vi "Shell and Tube Heat Exchanger 3.vi"() -> ()   [LabVIEW 2017]
uses:
  <vilib>/addons/control/pid/pid.llb/PID Control Input Filter (DBL).vi
  <vilib>/addons/control/pid/pid.llb/PID Advanced (DBL).vi
  <vilib>/addons/control/pid/NI_PID_pid.lvlib
panel:
  out "Makeup Flowrate":dbl caption="L/min"
  out "Makeup Temperature":dbl caption="C"
  in  "Pump Switch":bool
  out "Water Outlet Temperature":dbl=22.816489944987293 format="%.1f"
  in  "Flowrate Setpoint (GPM)":dbl=40.0 min=0.0 max=50.0 format="%.2f"
  out "Water Flowrate":dbl=-0.0005338564515105265 format="%.2f"
  out "Flow Control Valve":dbl(slide)=100.0 scale=0.0..100.0
  in  "Manual Control Override (Flow)":bool=TRUE
  in  "Set Manual Valve Position (Flow)":dbl(slide)=100.0 scale=0.0..100.0
  in  "Level Setpoint (ft)":dbl=1.5 min=0.0 max=2.0 format="%.2f"
  out "Liquid Level in Tank":dbl=-0.5117058749718749 format="%.2f"
  out "Level Control Valve":dbl(slide)=0.045055175643920364 scale=0.0..100.0
  in  "Manual Control Override (Level)":bool=TRUE
  in  "Set Manual Valve Position (Level)":dbl(slide) scale=0.0..100.0
  in  "stop":bool
  in  "Kc (Flow)":dbl=0.74
  in  "Ti (Flow)":dbl=0.036 caption="(min)"
  in  "Td (Flow)":dbl caption="(min)"
  in  "Kc (Level)":dbl=-75.0
  in  "Ti (Level)":dbl=0.005 caption="(min)"
  in  "Td (Level)":dbl caption="(min)"
  out "House Steam Pressure":dbl=-37.74410859375 caption="psig" format="%#.6g"
  out "Tube-Side Pressure Drop":dbl=-3.6907662628125 caption="psig"
  in  "Main Power":bool
  out "Water Feed Temperature":dbl=19.10777415276108 caption="C"
  in  "Steam Pressure Setpoint (psig)":dbl=10.0 min=0.0 max=45.0 format="%.2f"
  out "Steam Pressure":dbl=-38.330115825 caption="psig" format="%.2f"
  out "Steam Valve":dbl(slide) scale=0.0..100.0
  in  "Manual Control Override (Steam Pressure)":bool
  in  "Set Manual Valve Position (Steam Pressure)":dbl(slide) scale=0.0..100.0
  in  "Kc (Steam)":dbl=0.5
  in  "Ti (Steam)":dbl=0.05 caption="(min)"
  in  "Td (Steam)":dbl caption="(min)"
  out "Data Point Count":i32
  in  "Specify Time between Data Points (sec)":dbl=1.0
  in  "Cancel Data Collection":bool
  in  "Specify number of data points":i16=1
  in  "Enable 5":bool
  out "Saving Data 5":bool
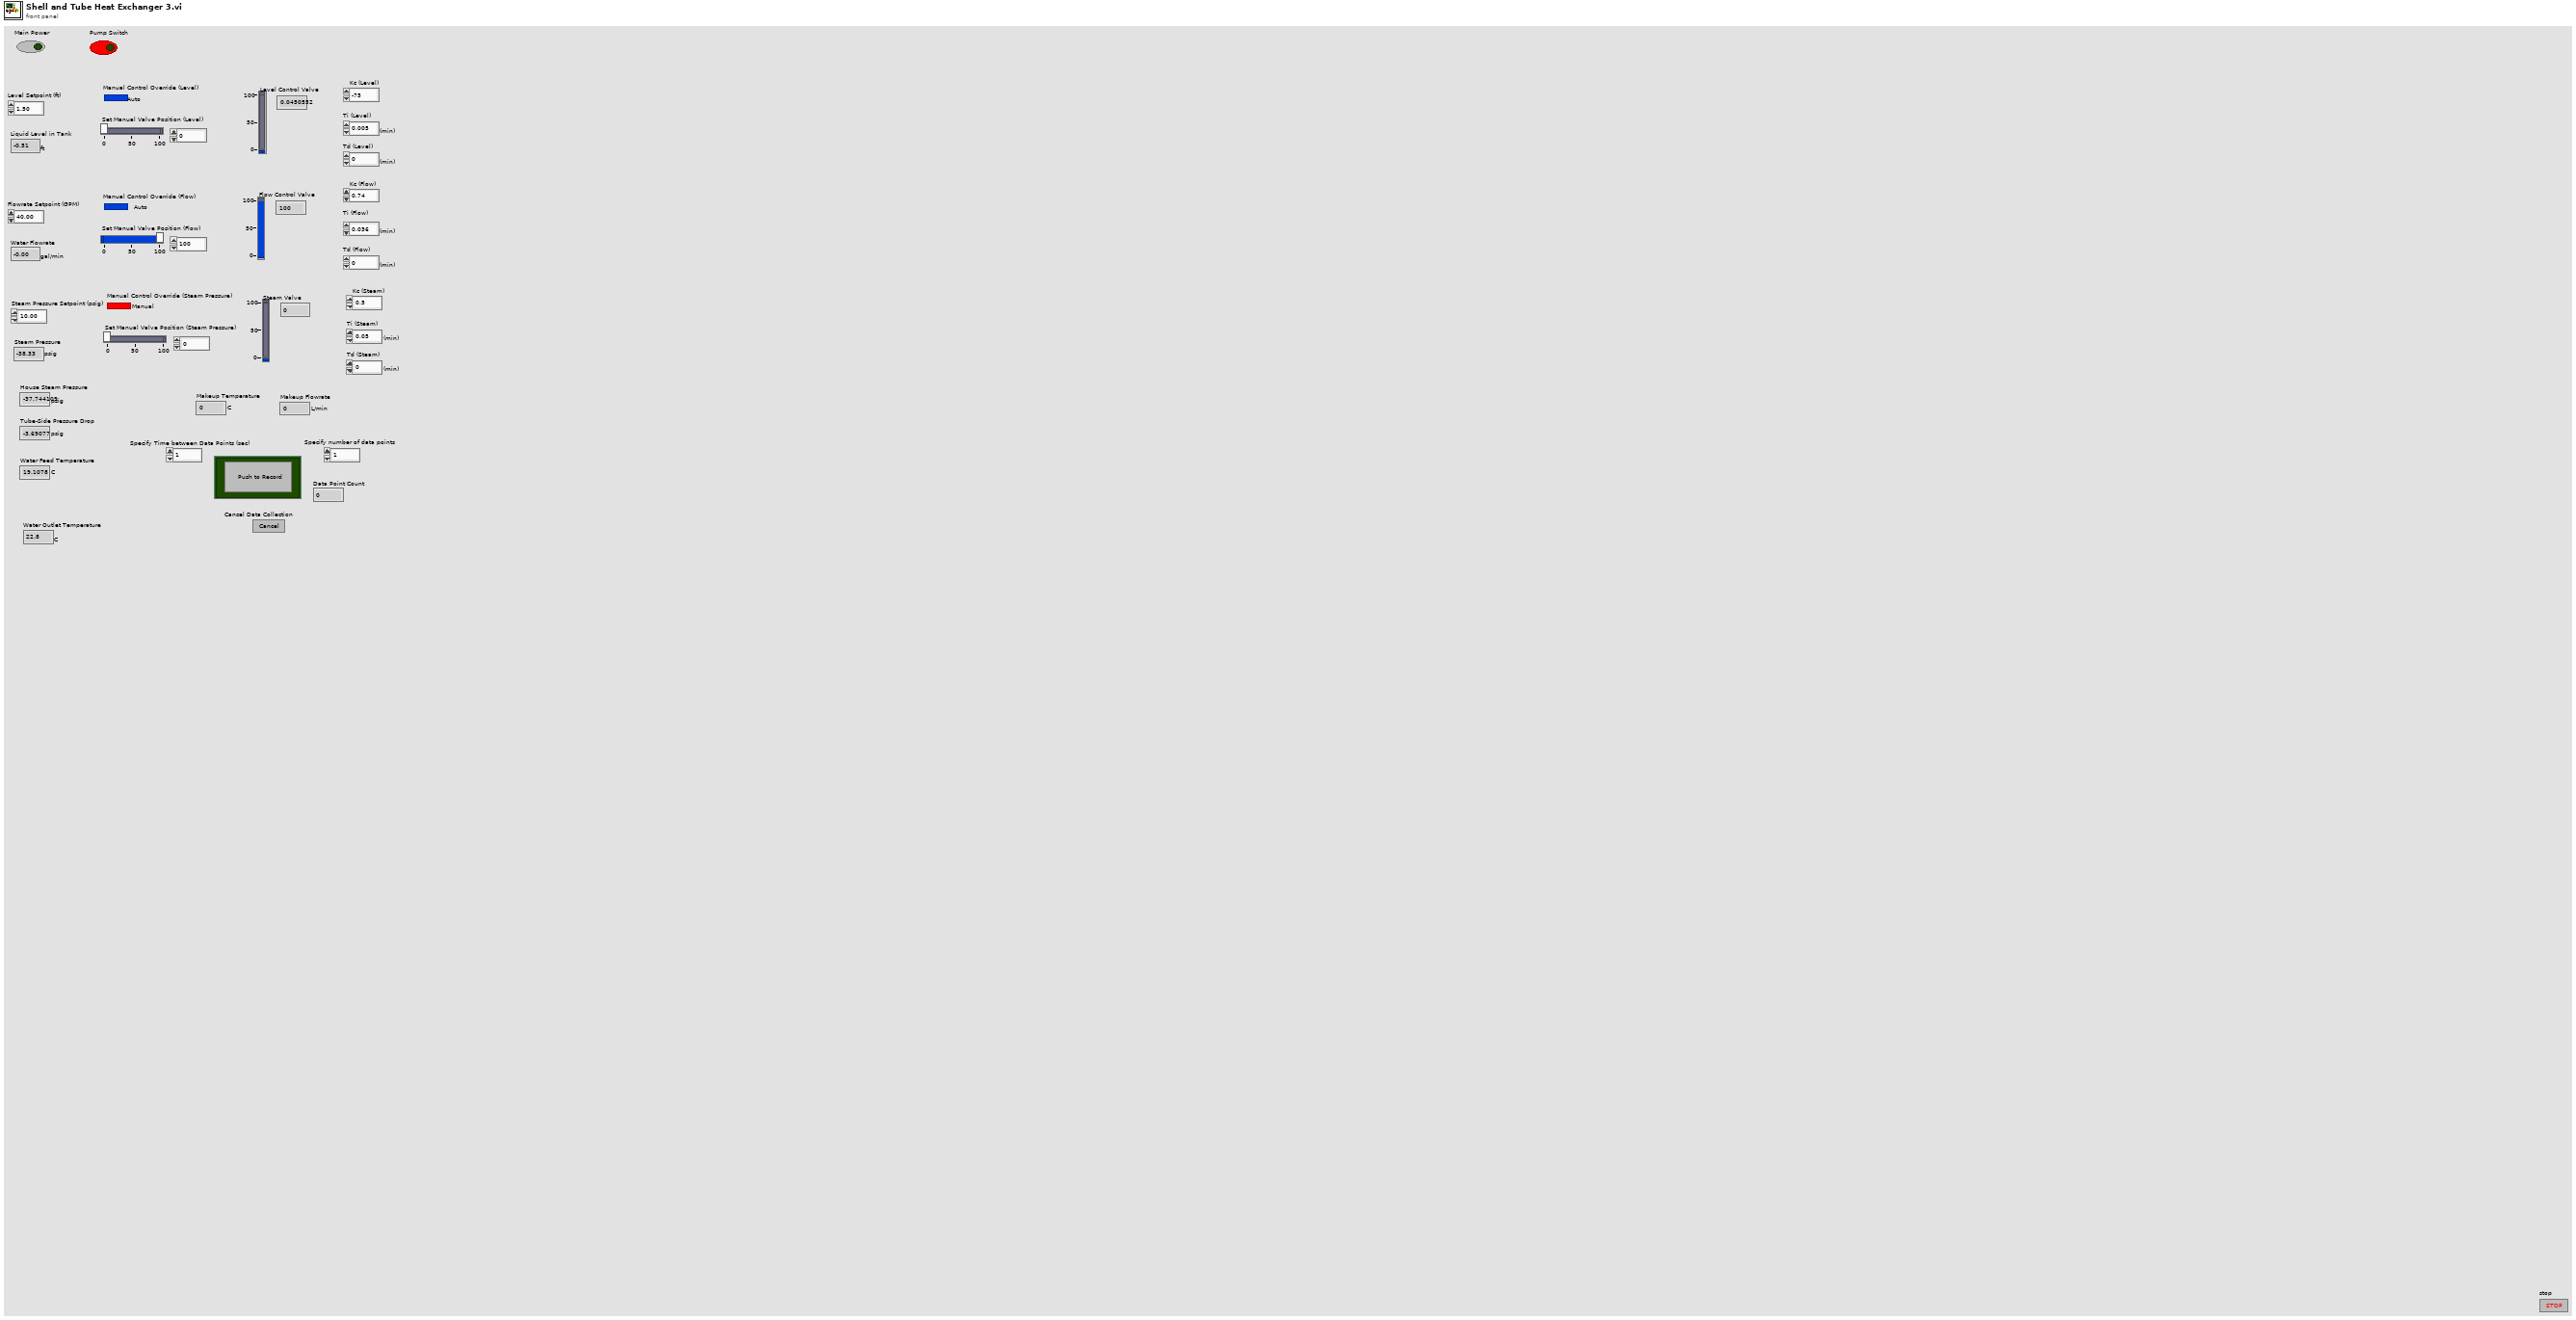
[diagram p1: front panel]
types:
  T1 = cluster{"Kc (Flow)":dbl, "Ti (Flow)":dbl, "Td (Flow)":dbl}
  T2 = cluster{"Kc (Level)":dbl, "Ti (Level)":dbl, "Td (Level)":dbl}
  T3 = cluster{"Kc (Steam)":dbl, "Ti (Steam)":dbl, "Td (Steam)":dbl}
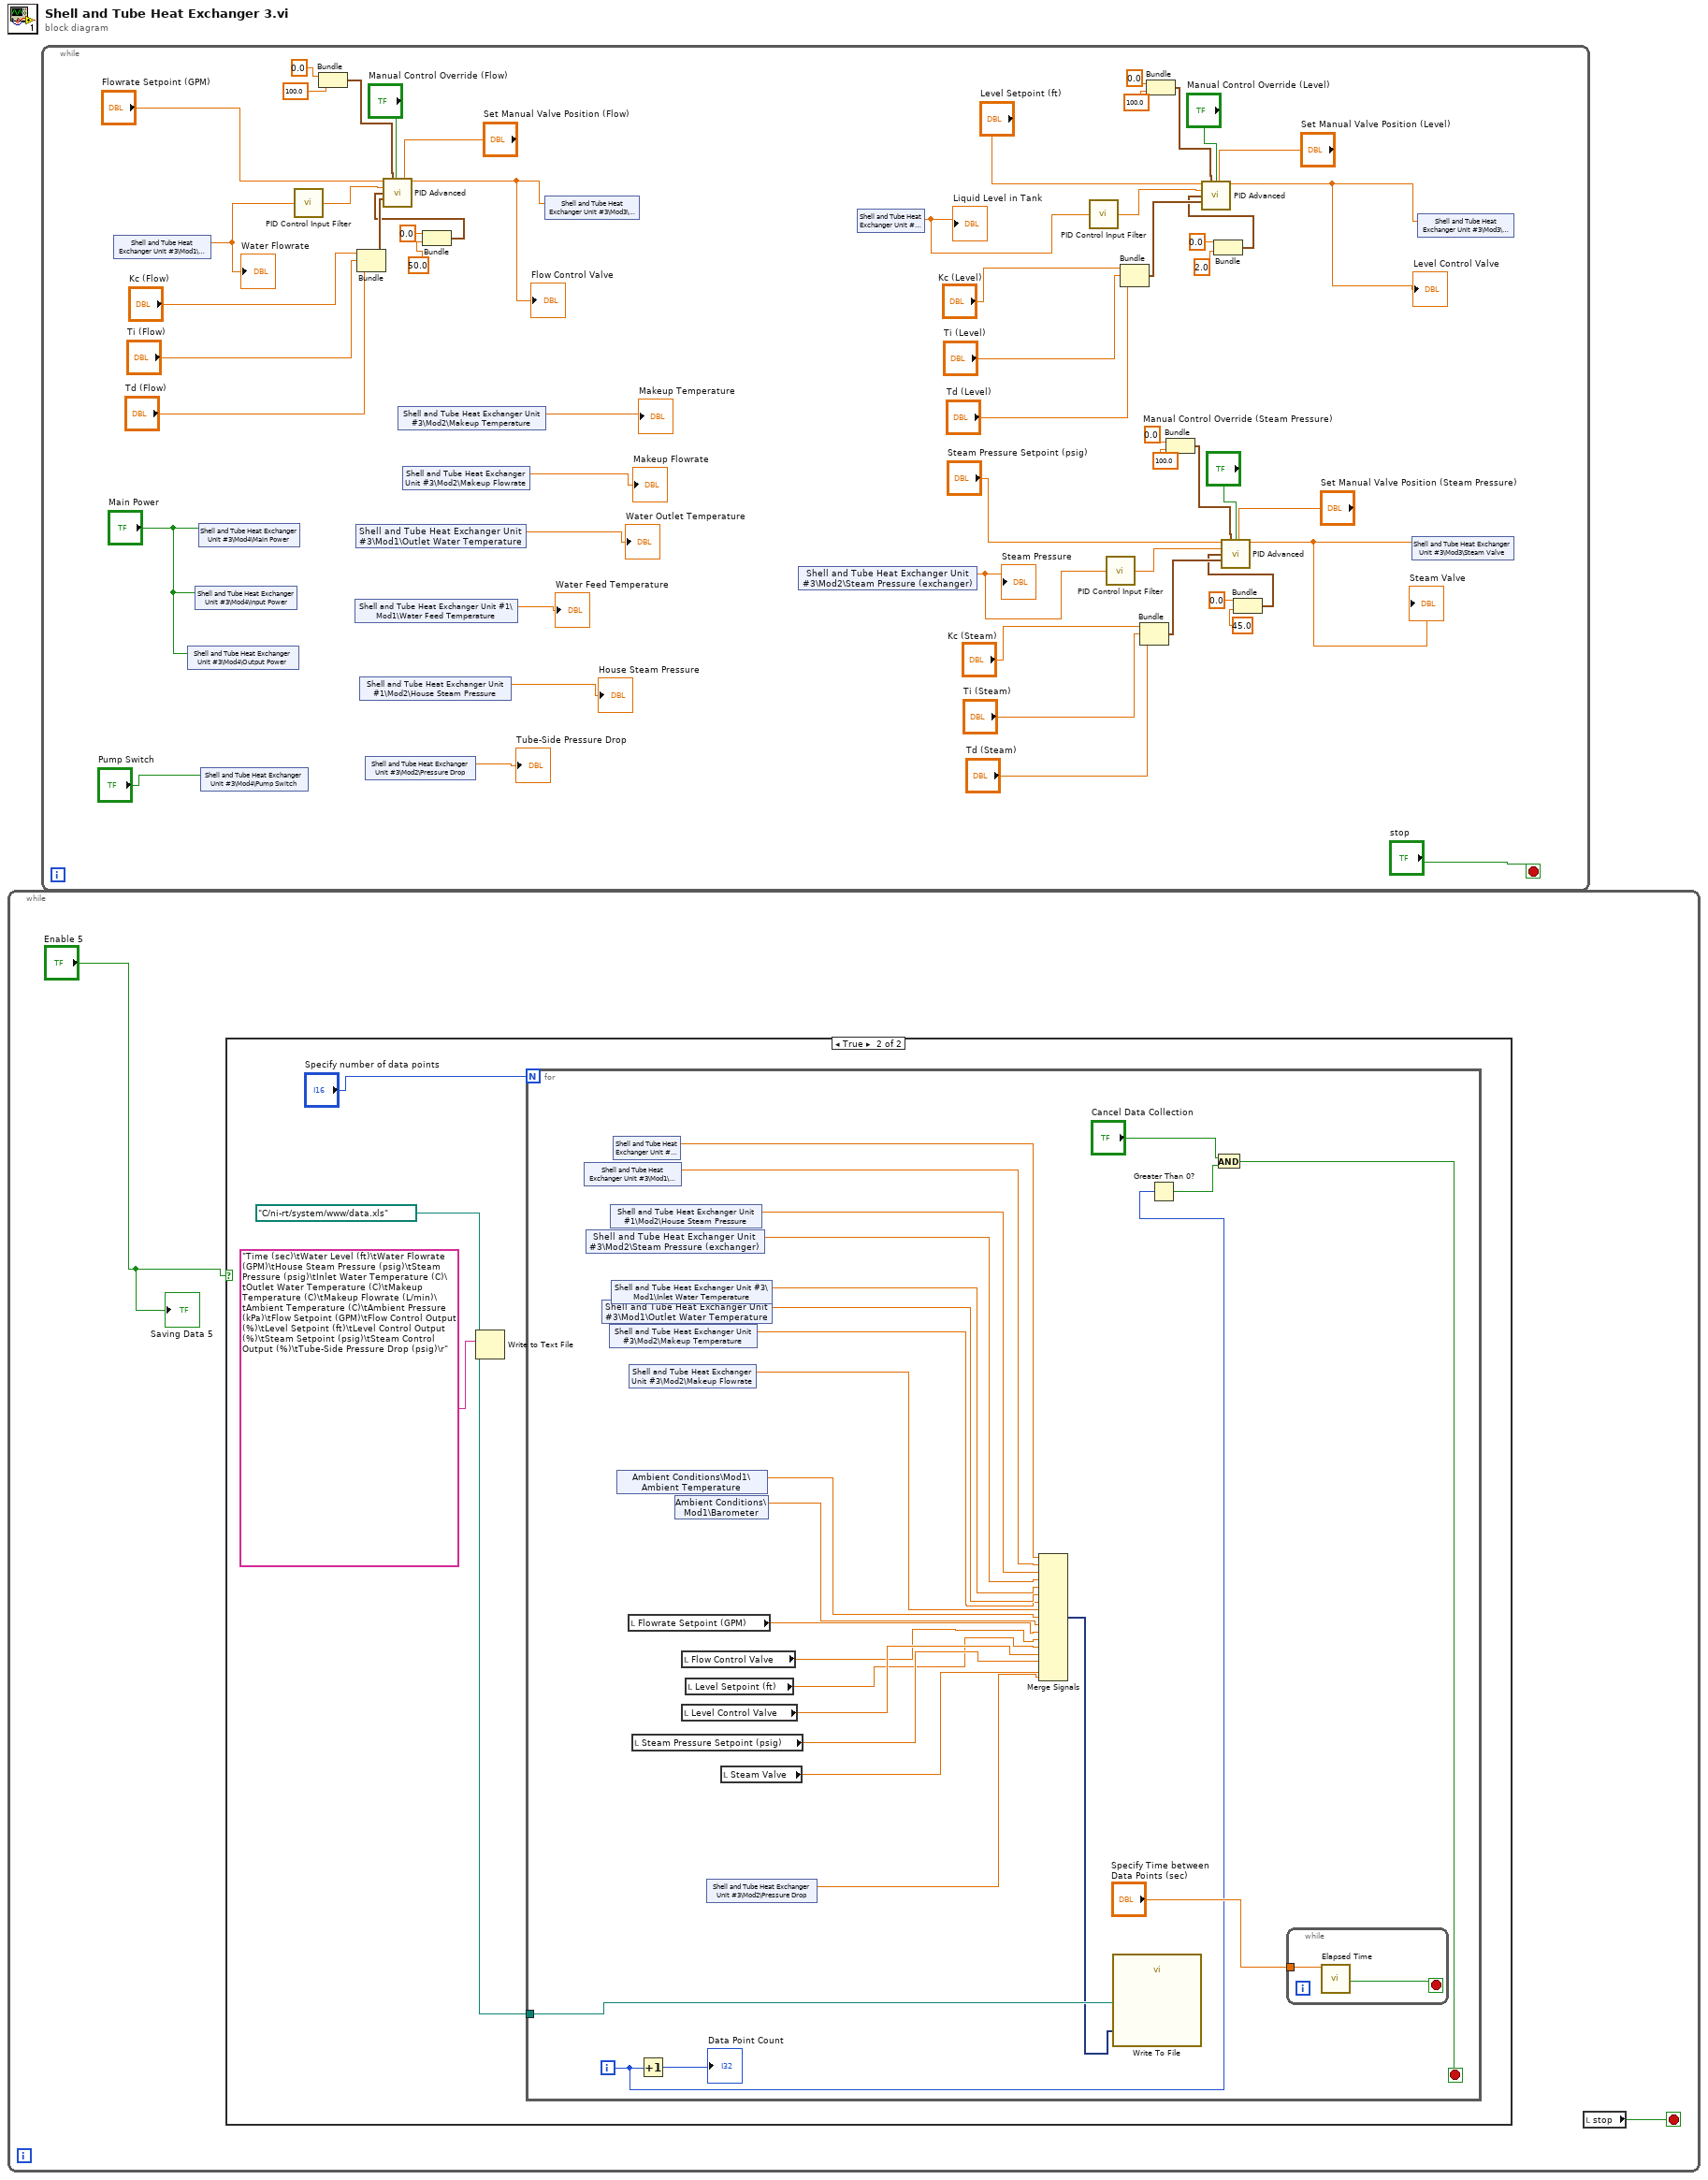
[diagram p0: block diagram]
diagram:
  n1 = while {
    stop <- w1 stop-if-true
    n2 = case shown="True" "Enable 5" {
      frame False {
      }
      frame True {
        w4 = path "C:/ni-rt/system/www/data.xls" ("Filename")
        n3 = Write to Text File(file (use dialog)=w4, text="Time (sec)\tWater Level (ft)\tWater Flowrate (GPM)\tHouse Steam Pressure (psig)\tSteam Pressure (psig)\tInlet Water Temperature (C)\tOutlet Water Temperature (C)\tMakeup Temperature (C)\tMakeup Flowrate (L/min)\tAmbient Temperature (C)\tAmbient Pressure (kPa)\tFlow Setpoint (GPM)\tFlow Control Output (%)\tLevel Setpoint (ft)\tLevel Control Output (%)\tSteam Setpoint (psig)\tSteam Control Output (%)\tTube-Side Pressure Drop (psig)\r") -> ()  [unwired: 2 in, 3 out]
        n4 = for {
          N: "Specify number of data points" -> [_]
          tunnel: w4 -> [w30]
          i -> [w26]
          stop <- w16 stop-if-true
          n5 = shared-variable "Shell and Tube Heat Exchanger Unit #3\\Mod1\\Water Flow"() -> (w23:dbl)  [unwired: 1 in, 1 out]
          n6 = shared-variable "Shell and Tube Heat Exchanger Unit #3\\Mod2\\Steam Pressure (exchanger)"() -> (w21:dbl)  [unwired: 1 in, 1 out]
          n7 = shared-variable "Shell and Tube Heat Exchanger Unit #3\\Mod1\\Outlet Water Temperature"() -> (w19:dbl)  [unwired: 1 in, 1 out]
          n8 = shared-variable "Shell and Tube Heat Exchanger Unit #3\\Mod2\\Makeup Temperature"() -> (w18:dbl)  [unwired: 1 in, 1 out]
          n9 = shared-variable "Shell and Tube Heat Exchanger Unit #1\\Mod2\\House Steam Pressure"() -> (w22:dbl)  [unwired: 1 in, 1 out]
          n10 = shared-variable "Shell and Tube Heat Exchanger Unit #3\\Mod1\\Inlet Water Temperature"() -> (w20:dbl)  [unwired: 1 in, 1 out]
          n11 = shared-variable "Shell and Tube Heat Exchanger Unit #3\\Mod2\\Level"() -> (w24:dbl)  [unwired: 1 in, 1 out]
          n12 = shared-variable "Ambient Conditions\\Mod1\\Ambient Temperature"() -> (w7:dbl)  [unwired: 1 in, 1 out]
          n13 = local read "Flowrate Setpoint (GPM)"() -> (w9:dbl)
          n14 = shared-variable "Shell and Tube Heat Exchanger Unit #3\\Mod2\\Makeup Flowrate"() -> (w6:dbl)  [unwired: 1 in, 1 out]
          n15 = local read "Steam Pressure Setpoint (psig)"() -> (w13:dbl)
          n16 = Increment(x=w26) -> (x+1=→"Data Point Count":i32)
          n17 = shared-variable "Ambient Conditions\\Mod1\\Barometer"() -> (w8:dbl)  [unwired: 1 in, 1 out]
          n18 = local read "Flow Control Valve"() -> (w10:dbl)
          n19 = local read "Level Control Valve"() -> (w12:dbl)
          n20 = local read "Level Setpoint (ft)"() -> (w11:dbl)
          n21 = shared-variable "Shell and Tube Heat Exchanger Unit #3\\Mod2\\Pressure Drop"() -> (w15:dbl)  [unwired: 1 in, 1 out]
          n22 = local read "Steam Valve"() -> (w14:dbl)
          n23 = Merge Signals(w24, w23, w22, w21, w20, w19, w18, w6, w7, w8, w9, w10, w11, w12, w13, w14, w15) -> (w28:dynamicdata)
          n24 = call "Write To File"("Signals"=w28, "Filename"=w30) -> ()  [unwired: 15 in, 3 out]
          n25 = Greater Than 0?(x=w26) -> (x > 0?=w25:bool)
          n26 = And(x="Cancel Data Collection", y=w25) -> (x .and. y?=w16:bool)
          n27 = while {
            tunnel: "Specify Time between Data Points (sec)" -> [w31]
            stop <- w32 stop-if-true
            n28 = call "Elapsed Time"("Time Target (s)"=w31) -> ("Time has Elapsed"=w32:bool)  [unwired: 11 in, 7 out]
          }
        }
      }
    }
    n29 = local read "stop"() -> (w1:bool)
    "Saving Data 5" <- "Enable 5"
  }
  n30 = while {
    stop <- "stop" stop-if-true
    n31 = shared-variable "Shell and Tube Heat Exchanger Unit #3\\Mod1\\Water Flow"() -> (w45:dbl)  [unwired: 1 in, 1 out]
    "Water Flowrate" <- w45
    n32 = shared-variable "Shell and Tube Heat Exchanger Unit #3\\Mod4\\Output Power"("Main Power") -> ()  [unwired: 1 in, 1 out]
    n33 = shared-variable "Shell and Tube Heat Exchanger Unit #3\\Mod4\\Input Power"("Main Power") -> ()  [unwired: 1 in, 1 out]
    n34 = shared-variable "Shell and Tube Heat Exchanger Unit #3\\Mod4\\Main Power"("Main Power") -> ()  [unwired: 1 in, 1 out]
    n35 = shared-variable "Shell and Tube Heat Exchanger Unit #3\\Mod4\\Pump Switch"("Pump Switch") -> ()  [unwired: 1 in, 1 out]
    n36 = call-poly <vilib>:"PID Control Input Filter.vi"("input"=w45) -> ("output"=w44:dbl)  [unwired: 4 in]
    n37 = Bundle(0.0, 100.0) -> (w70:cluster{dbl, dbl})  [unwired: 1 in]
    n38 = shared-variable "Shell and Tube Heat Exchanger Unit #1\\Mod1\\Water Feed Temperature"() -> (→"Water Feed Temperature":dbl)  [unwired: 1 in, 1 out]
    n39 = shared-variable "Shell and Tube Heat Exchanger Unit #3\\Mod1\\Outlet Water Temperature"() -> (→"Water Outlet Temperature":dbl)  [unwired: 1 in, 1 out]
    n40 = Bundle("Kc (Flow)"="Kc (Flow)", "Ti (Flow)"="Ti (Flow)", "Td (Flow)"="Td (Flow)") -> (w85:T1)  [unwired: 1 in]
    n41 = shared-variable "Shell and Tube Heat Exchanger Unit #1\\Mod2\\House Steam Pressure"() -> (→"House Steam Pressure":dbl)  [unwired: 1 in, 1 out]
    n42 = shared-variable "Shell and Tube Heat Exchanger Unit #3\\Mod2\\Pressure Drop"() -> (→"Tube-Side Pressure Drop":dbl)  [unwired: 1 in, 1 out]
    n43 = shared-variable "Shell and Tube Heat Exchanger Unit #3\\Mod2\\Makeup Temperature"() -> (→"Makeup Temperature":dbl)  [unwired: 1 in, 1 out]
    n44 = shared-variable "Shell and Tube Heat Exchanger Unit #3\\Mod2\\Makeup Flowrate"() -> (→"Makeup Flowrate":dbl)  [unwired: 1 in, 1 out]
    n45 = Bundle(0.0, 50.0) -> (w67:cluster{dbl, dbl})  [unwired: 1 in]
    n46 = call-poly <vilib>:"PID Advanced.vi"("setpoint"="Flowrate Setpoint (GPM)", "output range"=w70, "auto? (T)"="Manual Control Override (Flow)", "manual control"="Set Manual Valve Position (Flow)", "process variable"=w44, "setpoint range"=w67, "PID gains"=w85) -> ("output"=w39:dbl)  [unwired: 7 in, 1 out]
    "Flow Control Valve" <- w39
    n47 = shared-variable "Shell and Tube Heat Exchanger Unit #3\\Mod3\\Flow Valve"(w39) -> ()  [unwired: 1 in, 1 out]
    n48 = shared-variable "Shell and Tube Heat Exchanger Unit #3\\Mod2\\Steam Pressure (exchanger)"() -> (w43:dbl)  [unwired: 1 in, 1 out]
    "Steam Pressure" <- w43
    n49 = shared-variable "Shell and Tube Heat Exchanger Unit #3\\Mod2\\Level"() -> (w47:dbl)  [unwired: 1 in, 1 out]
    "Liquid Level in Tank" <- w47
    n50 = call-poly <vilib>:"PID Control Input Filter.vi"("input"=w47) -> ("output"=w46:dbl)  [unwired: 4 in]
    n51 = call-poly <vilib>:"PID Control Input Filter.vi"("input"=w43) -> ("output"=w42:dbl)  [unwired: 4 in]
    n52 = Bundle("Kc (Level)"="Kc (Level)", "Ti (Level)"="Ti (Level)", "Td (Level)"="Td (Level)") -> (w87:T2)  [unwired: 1 in]
    n53 = Bundle("Kc (Steam)"="Kc (Steam)", "Ti (Steam)"="Ti (Steam)", "Td (Steam)"="Td (Steam)") -> (w58:T3)  [unwired: 1 in]
    n54 = Bundle(0.0, 100.0) -> (w73:cluster{dbl, dbl})  [unwired: 1 in]
    n55 = Bundle(0.0, 100.0) -> (w53:cluster{dbl, dbl})  [unwired: 1 in]
    n56 = Bundle(0.0, 2.0) -> (w64:cluster{dbl, dbl})  [unwired: 1 in]
    n57 = call-poly <vilib>:"PID Advanced.vi"("setpoint"="Level Setpoint (ft)", "output range"=w73, "auto? (T)"="Manual Control Override (Level)", "manual control"="Set Manual Valve Position (Level)", "process variable"=w46, "setpoint range"=w64, "PID gains"=w87) -> ("output"=w38:dbl)  [unwired: 7 in, 1 out]
    "Level Control Valve" <- w38
    n58 = Bundle(0.0, 45.0) -> (w50:cluster{dbl, dbl})  [unwired: 1 in]
    n59 = call-poly <vilib>:"PID Advanced.vi"("setpoint"="Steam Pressure Setpoint (psig)", "output range"=w53, "auto? (T)"="Manual Control Override (Steam Pressure)", "manual control"="Set Manual Valve Position (Steam Pressure)", "process variable"=w42, "setpoint range"=w50, "PID gains"=w58) -> ("output"=w36:dbl)  [unwired: 7 in, 1 out]
    "Steam Valve" <- w36
    n60 = shared-variable "Shell and Tube Heat Exchanger Unit #3\\Mod3\\Steam Valve"(w36) -> ()  [unwired: 1 in, 1 out]
    n61 = shared-variable "Shell and Tube Heat Exchanger Unit #3\\Mod3\\Level Valve"(w38) -> ()  [unwired: 1 in, 1 out]
  }
